vi "SMTP Email Send Multiple Attachments.vi"(0 "recipients":string[](array[string]), 1 "mail server":string, 2 "return address":string, 5 "subject ([No Subject])":string="[No Subject]", 7 "message":string, 9 "attachments":T1(array[cluster]), 11 "error in (no error)":errorcluster) -> (4 "invalid recipients":string[](array[string]), 15 "error out":errorcluster)   [LabVIEW 2009, in "NewNI_SMTPEmail.lvlib"]
doc: "Sends an email with multiple file and data attachments to a list of recipients."
uses:
  NewNI_SMTPEmail.lvlib
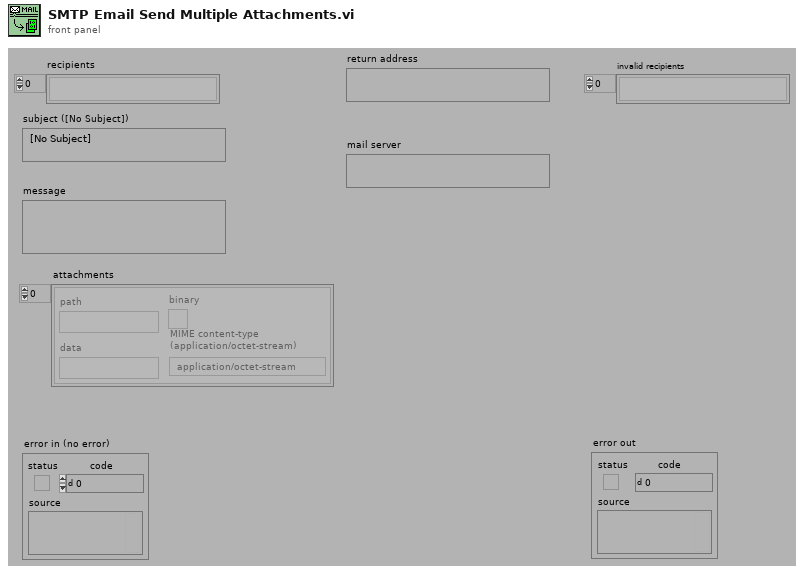
[diagram p1: front panel]
types:
  T1 = cluster{"path":path, "data":string, "binary":bool, "MIME content-type \n(application/octet-stream)":string}[]
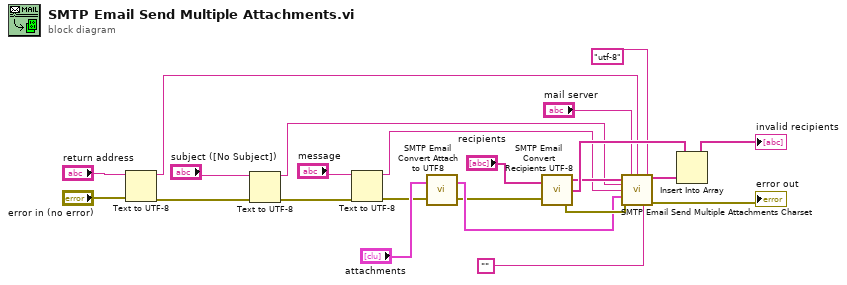
[diagram p0: block diagram]
diagram:
  n1 = Text to UTF-8(8:"error in (no error)", 11:"return address") -> (0:w19:errorcluster, 3:w10:string)
  n2 = Text to UTF-8(8:w19, 11:"subject ([No Subject])") -> (0:w21:errorcluster, 3:w8:string)
  n3 = Text to UTF-8(8:w21, 11:"message") -> (0:w3:errorcluster, 3:w7:string)
  n4 = call "SMTP Email Convert Attach to UTF8.vi"("error in"=w3, "attachments"="attachments") -> ("error out"=w2:errorcluster, "UTF-8 Attachments"=w4:T1)
  n5 = call "SMTP Email Convert Recipients UTF-8.vi"("recipients"="recipients", "error in"=w2) -> ("convertible recipients"=w12:string[], "unconvertible recipients"=w13:string[], "error out"=w16:errorcluster)
  n6 = call "SMTP Email Send Multiple Attachments Charset.vi"("recipients"=w12, "mail server"="mail server", "return address"=w10, "character set (us-ascii)"="utf-8", "subject ([No Subject])"=w8, "message"=w7, "attachments"=w4, "error in (no error)"=w16, "translit"="") -> ("invalid recipients"=w17:string[], "error out"=→"error out":errorcluster)  [unwired: 1 in, 4 out]
  n7 = Insert Into Array(array=w13, new element=w17) -> (→"invalid recipients":string[])  [unwired: 1 in]
